vi "TempGraficoWhile.vi"() -> ()   [LabVIEW 2017]
panel:
  out "Valor x Amostras":dbl(graph)
  in  "Escala":bool
  in  "Chave":bool
  # "On"
  # "ºF"
  # "Off"
  # "ºC"
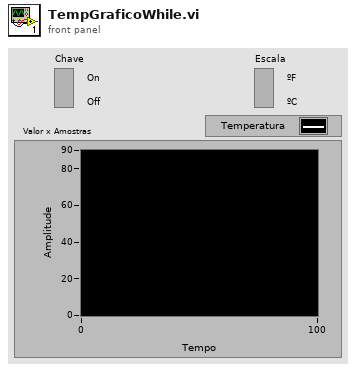
[diagram p1: front panel]
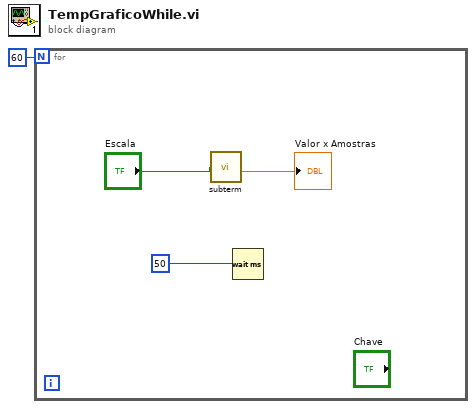
[diagram p0: block diagram]
diagram:
  n1 = for {
    N: 60 -> [_]
    n2 = call "subterm.vi"("Escala"="Escala") -> ("Temperatura"=→"Valor x Amostras":dbl)
    n3 = Wait (ms)(milliseconds to wait=50) -> ()  [unwired: 1 out]
  }
